vi "Func-엑셀 데이터를 그래프로 출력.vi"() -> ()   [LabVIEW 2015] (continued)
\n740.23\n740.24\n740.26\n740.28\n740.29\n740.31\n740.33\n740.34\n740.36\n740.38\n740.4\n740.41\n740.43\n740.44\n740.46\n740.48\n740.5\n740.51\n740.53\n740.54\n740.56\n740.58\n740.59\n740.61\n740.63\n740.65\n740.66\n740.68\n740.69\n740.71\n740.73\n740.74\n740.76\n740.78\n740.79\n740.81\n740.83\n740.84\n740.86\n740.88\n740.89\n740.91\n740.93\n740.94\n740.96\n740.98\n740.99\n741.01\n741.03\n741.04\n741.06\n741.08\n741.09\n741.11\n741.13\n741.14\n741.16\n741.18\n741.2\n741.21\n741.23\n741.24\n741.26\n741.28\n741.29\n741.31\n741.33\n741.34\n741.36\n741.38\n741.39\n741.41\n741.43\n741.44\n741.46\n741.48\n741.49\n741.51\n741.53\n741.54\n741.56\n741.58\n741.59\n741.61\n741.63\n741.64\n741.66\n741.68\n741.7\n741.71\n741.73\n741.74\n741.76\n741.78\n741.79\n741.81\n741.83\n741.84\n741.86\n741.88\n741.89\n741.91\n741.93\n741.94\n741.96\n741.98\n741.99\n742.01\n742.03\n742.04\n742.06\n742.08\n742.09\n742.11\n742.13\n742.14\n742.16\n742.18\n742.19\n742.21\n742.23\n742.24\n742.26\n742.28\n742.29\n742.31\n742.33\n742.34\n742.36\n742.38\n742.39\n742.41\n742.43\n742.44\n742.46\n742.48\n742.49\n742.51\n742.53\n742.54\n742.56\n742.58\n742.59\n742.61\n742.63\n742.64\n742.66\n742.68\n742.69\n742.71\n742.73\n742.74\n742.76\n742.78\n742.8\n742.81\n742.83\n742.84\n742.86\n742.88\n742.89\n742.91\n742.93\n742.94\n742.96\n742.98\n742.99\n743.01\n743.03\n743.04\n743.06\n743.08\n743.09\n743.11\n743.13\n743.15\n743.16\n743.18\n743.19\n743.21\n743.23\n743.25\n743.26\n743.28\n743.29\n743.31\n743.33\n743.34\n743.36\n743.38\n743.39\n743.41\n743.43\n743.44\n743.46\n743.48\n743.5\n743.51\n743.53\n743.54\n743.56\n743.58\n743.6\n743.61\n743.63\n743.64\n743.66\n743.68\n743.69\n743.71\n743.73\n743.74\n743.76\n743.78\n743.79\n743.81\n743.83\n743.84\n743.86\n743.88\n743.89\n743.91\n743.93\n743.95\n743.96\n743.98\n743.99\n744.01\n744.03\n744.04\n744.06\n744.08\n744.09\n744.11\n744.13\n744.14\n744.16\n744.18\n744.19\n744.21\n744.23\n744.24\n744.26\n744.28\n744.3\n744.31\n744.33\n744.34\n744.36\n744.38\n744.39\n744.41\n744.43\n744.44\n744.46\n744.48\n744.49\n744.51\n744.53\n744.54\n744.56\n744.58\n744.59\n744.61\n744.63\n744.64\n744.66\n744.68\n744.69\n744.71\n744.73\n744.74\n744.76\n744.78\n744.79\n744.81\n744.83\n744.84\n744.86\n744.88\n744.89\n744.91\n744.93\n744.94\n744.96\n744.98\n744.99\n745.01\n745.03\n745.04\n745.06\n745.08\n745.09\n745.11\n745.13\n745.14\n745.16\n745.18\n745.19\n745.21\n745.23\n745.24\n745.26\n745.28\n745.29\n745.31\n745.33\n745.34\n745.36\n745.38\n745.39\n745.41\n745.43\n745.44\n745.46\n745.48\n745.49\n745.51\n745.53\n745.54\n745.56\n745.58\n745.59\n745.61\n745.63\n745.64\n745.66\n745.68\n745.69\n745.71\n745.73\n745.74\n745.76\n745.78\n745.79\n745.81\n745.83\n745.84\n745.86\n745.88\n745.89\n745.91\n745.93\n745.94\n745.96\n745.98\n745.99\n746.01\n746.03\n746.04\n746.06\n746.08\n746.09\n746.11\n746.13\n746.14\n746.16\n746.18\n746.19\n746.21\n746.23\n746.25\n746.26\n746.28\n746.29\n746.31\n746.33\n746.34\n746.36\n746.38\n746.39\n746.41\n746.43\n746.44\n746.46\n746.48\n746.5\n746.51\n746.53\n746.54\n746.56\n746.58\n746.6\n746.61\n746.63\n746.64\n746.66\n746.68\n746.69\n746.71\n746.73\n746.74\n746.76\n746.78\n746.79\n746.81\n746.83\n746.84\n746.86\n746.88\n746.89\n746.91\n746.93\n746.94\n746.96\n746.98\n746.99\n747.01\n747.03\n747.05\n747.06\n747.08\n747.09\n747.11\n747.13\n747.14\n747.16\n747.18\n747.19\n747.21\n747.23\n747.24\n747.26\n747.28\n747.29\n747.31\n747.33\n747.34\n747.36\n747.38\n747.39\n747.41\n747.43\n747.44\n747.46\n747.48\n747.49\n747.51\n747.53\n747.54\n747.56\n747.58\n747.59\n747.61\n747.63\n747.64\n747.66\n747.68\n747.69\n747.71\n747.73\n747.74\n747.76\n747.78\n747.79\n747.81\n747.83\n747.84\n747.86\n747.88\n747.9\n747.91\n747.93\n747.94\n747.96\n747.98\n747.99\n748.01\n748.03\n748.04\n748.06\n748.08\n748.09\n748.11\n748.13\n748.14\n748.16\n748.18\n748.19\n748.21\n748.23\n748.24\n748.26\n748.28\n748.29\n748.31\n748.33\n748.34\n748.36\n748.38\n748.39\n748.41\n748.43\n748.44\n748.46\n748.48\n748.49\n748.51\n748.53\n748.54\n748.56\n748.58\n748.59\n748.61\n748.63\n748.64\n748.66\n748.68\n748.69\n748.71\n748.73\n748.74\n748.76\n748.78\n748.79\n748.81\n748.83\n748.84\n748.86\n748.88\n748.89\n748.91\n748.93\n748.94\n748.96\n748.98\n749\n749.01\n749.03\n749.04\n749.06\n749.08\n749.09\n749.11\n749.13\n749.14\n749.16\n749.18\n749.19\n749.21\n749.23\n749.24\n749.26\n749.28\n749.29\n749.31\n749.33\n749.35\n749.36\n749.38\n749.39\n749.41\n749.43\n749.44\n749.46\n749.48\n749.49\n749.51\n749.53\n749.54\n749.56\n749.58\n749.6\n749.61\n749.63\n749.64\n749.66\n749.68\n749.7\n749.71\n749.73\n749.74\n749.76\n749.78\n749.79\n749.81\n749.83\n749.85\n749.86\n749.88\n749.89\n749.91\n749.93\n749.95\n749.96\n749.98\n749.99\n750.01\n750.03\n750.05\n750.06\n750.08\n750.09\n750.11\n750.13\n750.14\n750.16\n750.18\n750.19\n750.21\n750.23\n750.24\n750.26\n750.28\n750.3\n750.31\n750.33\n750.34\n750.36\n750.38\n750.39\n750.41\n750.43\n750.44\n750.46\n750.48\n750.49\n750.51\n750.53\n750.54\n750.56\n750.58\n750.59\n750.61\n750.63\n750.64\n750.66\n750.68\n750.69\n750.71\n750.73\n750.74\n750.76\n750.78\n750.79\n750.81\n750.83\n750.84\n750.86\n750.88\n750.89\n750.91\n750.93\n750.94\n750.96\n750.98\n750.99\n751.01\n751.03\n751.04\n751.06\n751.08\n751.09\n751.11\n751.13\n751.14\n751.16\n751.18\n751.19\n751.21\n751.23\n751.24\n751.26\n751.28\n751.29\n751.31\n751.33\n751.34\n751.36\n751.38\n751.39\n751.41\n751.43\n751.44\n751.46\n751.48\n751.49\n751.51\n751.53\n751.54\n751.56\n751.58\n751.59\n751.61\n751.63\n751.64\n751.66\n751.68\n751.69\n751.71\n751.73\n751.74\n751.76\n751.78\n751.79\n751.81\n751.83\n751.84\n751.86\n751.88\n751.89\n751.91\n751.93\n751.94\n751.96\n751.98\n751.99\n752.01\n752.03\n752.04\n752.06\n752.08\n752.1\n752.11\n752.13\n752.14\n752.16\n752.18\n752.19\n752.21\n752.23\n752.24\n752.26\n752.28\n752.29\n752.31\n752.33\n752.35\n752.36\n752.38\n752.39\n752.41\n752.43\n752.45\n752.46\n752.48\n752.49\n752.51\n752.53\n752.54\n752.56\n752.58\n752.59\n752.61\n752.63\n752.64\n752.66\n752.68\n752.7\n752.71\n752.73\n752.74\n752.76\n752.78\n752.8\n752.81\n752.83\n752.84\n752.86\n752.88\n752.89\n752.91\n752.93\n752.94\n752.96\n752.98\n752.99\n753.01\n753.03\n753.05\n753.06\n753.08\n753.09\n753.11\n753.13\n753.14\n753.16\n753.18\n753.19\n753.21\n753.23\n753.24\n753.26\n753.28\n753.29\n753.31\n753.33\n753.34\n753.36\n753.38\n753.4\n753.41\n753.43\n753.44\n753.46\n753.48\n753.49\n753.51\n753.53\n753.54\n753.56\n753.58\n753.59\n753.61\n753.63\n753.65\n753.66\n753.68\n753.69\n753.71\n753.73\n753.75\n753.76\n753.78\n753.79\n753.81\n753.83\n753.84\n753.86\n753.88\n753.89\n753.91\n753.93\n753.95\n753.96\n753.98\n753.99\n754.01\n754.03\n754.04\n754.06\n754.08\n754.09\n754.11\n754.13\n754.14\n754.16\n754.18\n754.19\n754.21\n754.23\n754.24\n754.26\n754.28\n754.29\n754.31\n754.33\n754.34\n754.36\n754.38\n754.39\n754.41\n754.43\n754.44\n754.46\n754.48\n754.49\n754.51\n754.53\n754.54\n754.56\n754.58\n754.59\n754.61\n754.63\n754.64\n754.66\n754.68\n754.69\n754.71\n754.73\n754.74\n754.76\n754.78\n754.79\n754.81\n754.83\n754.84\n754.86\n754.88\n754.89\n754.91\n754.93\n754.94\n754.96\n754.98\n754.99\n755.01\n755.03\n755.04\n755.06\n755.08\n755.1\n755.11\n755.13\n755.14\n755.16\n755.18\n755.19\n755.21\n755.23\n755.24\n755.26\n755.28\n755.29\n755.31\n755.33\n755.34\n755.36\n755.38\n755.39\n755.41\n755.43\n755.45\n755.46\n755.48\n755.49\n755.51\n755.53\n755.54\n755.56\n755.58\n755.59\n755.61\n755.63\n755.64\n755.66\n755.68\n755.69\n755.71\n755.73\n755.74\n755.76\n755.78\n755.8\n755.81\n755.83\n755.84\n755.86\n755.88\n755.9\n755.91\n755.93\n755.94\n755.96\n755.98\n755.99\n756.01\n756.03\n756.05\n756.06\n756.08\n756.09\n756.11\n756.13\n756.14\n756.16\n756.18\n756.19\n756.21\n756.23\n756.24\n756.26\n756.28\n756.29\n756.31\n756.33\n756.34\n756.36\n756.38\n756.4\n756.41\n756.43\n756.44\n756.46\n756.48\n756.49\n756.51\n756.53\n756.54\n756.56\n756.58\n756.59\n756.61\n756.63\n756.65\n756.66\n756.68\n756.69\n756.71\n756.73\n756.74\n756.76\n756.78\n756.79\n756.81\n756.83\n756.84\n756.86\n756.88\n756.89\n756.91\n756.93\n756.94\n756.96\n756.98\n756.99\n757.01\n757.03\n757.04\n757.06\n757.08\n757.09\n757.11\n757.13\n757.14\n757.16\n757.18\n757.19\n757.21\n757.23\n757.24\n757.26\n757.28\n757.29\n757.31\n757.33\n757.34\n757.36\n757.38\n757.39\n757.41\n757.43\n757.44\n757.46\n757.48\n757.49\n757.51\n757.53\n757.54\n757.56\n757.58\n757.59\n757.61\n757.63\n757.64\n757.66\n757.68\n757.69\n757.71\n757.73\n757.74\n757.76\n757.78\n757.79\n757.81\n757.83\n757.84\n757.86\n757.88\n757.89\n757.91\n757.93\n757.94\n757.96\n757.98\n757.99\n758.01\n758.03\n758.04\n758.06\n758.08\n758.09\n758.11\n758.13\n758.14\n758.16\n758.18\n758.2\n758.21\n758.23\n758.24\n758.26\n758.28\n758.29\n758.31\n758.33\n758.34\n758.36\n758.38\n758.39\n758.41\n758.43\n758.44\n758.46\n758.48\n758.49\n758.51\n758.53\n758.55\n758.56\n758.58\n758.59\n758.61\n758.63\n758.64\n758.66\n758.68\n758.69\n758.71\n758.73\n758.74\n758.76\n758.78\n758.8\n758.81\n758.83\n758.84\n758.86\n758.88\n758.9\n758.91\n758.93\n758.94\n758.96\n758.98\n758.99\n759.01\n759.03\n759.04\n759.06\n759.08\n759.09\n759.11\n759.13\n759.15\n759.16\n759.18\n759.19\n759.21\n759.23\n759.25\n759.26\n759.28\n759.29\n759.31\n759.33\n759.34\n759.36\n759.38\n759.39\n759.41\n759.43\n759.44\n759.46\n759.48\n759.5\n759.51\n759.53\n759.54\n759.56\n759.58\n759.59\n759.61\n759.63\n759.64\n759.66\n759.68\n759.7\n759.71\n759.73\n759.74\n759.76\n759.78\n759.79\n759.81\n759.83\n759.84\n759.86\n759.88\n759.89\n759.91\n759.93\n759.94\n759.96\n759.98\n759.99\n760.01\n760.03\n760.04\n760.06\n760.08\n760.09\n760.11\n760.13\n760.14\n760.16\n760.18\n760.19\n760.21\n760.23\n760.24\n760.26\n760.28\n760.29\n760.31\n760.33\n760.34\n760.36\n760.38\n760.39\n760.41\n760.43\n760.44\n760.46\n760.48\n760.49\n760.51\n760.53\n760.54\n760.56\n760.58\n760.59\n760.61\n760.63\n760.64\n760.66\n760.68\n760.69\n760.71\n760.73\n760.74\n760.76\n760.78\n760.79\n760.81\n760.83\n760.84\n760.86\n760.88\n760.89\n760.91\n760.93\n760.94\n760.96\n760.98\n760.99\n761.01\n761.03\n761.04\n761.06\n761.08\n761.09\n761.11\n761.13\n761.14\n761.16\n761.18\n761.19\n761.21\n761.23\n761.24\n761.26\n761.28\n761.29\n761.31\n761.33\n761.34\n761.36\n761.38\n761.39\n761.41\n761.43\n761.44\n761.46\n761.48\n761.49\n761.51\n761.53\n761.54\n761.56\n761.58\n761.59\n761.61\n761.63\n761.65\n761.66\n761.68\n761.69\n761.71\n761.73\n761.74\n761.76\n761.78\n761.79\n761.81\n761.83\n761.84\n761.86\n761.88\n761.9\n761.91\n761.93\n761.94\n761.96\n761.98\n762\n762.01\n762.03\n762.04\n762.06\n762.08\n762.09\n762.11\n762.13\n762.14\n762.16\n762.18\n762.19\n762.21\n762.23\n762.25\n762.26\n762.28\n762.29\n762.31\n762.33\n762.34\n762.36\n762.38\n762.39\n762.41\n762.43\n762.45\n762.46\n762.48\n762.49\n762.51\n762.53\n762.54\n762.56\n762.58\n762.59\n762.61\n762.63\n762.64\n762.66\n762.68\n762.69\n762.71\n762.73\n762.74\n762.76\n762.78\n762.79\n762.81\n762.83\n762.84\n762.86\n762.88\n762.89\n762.91\n762.93\n762.95\n762.96\n762.98\n762.99\n763.01\n763.03\n763.04\n763.06\n763.08\n763.09\n763.11\n763.13\n763.14\n763.16\n763.18\n763.19\n763.21\n763.23\n763.24\n763.26\n763.28\n763.29\n763.31\n763.33\n763.34\n763.36\n763.38\n763.39\n763.41\n763.43\n763.44\n763.46\n763.48\n763.49\n763.51\n763.53\n763.54\n763.56\n763.58\n763.59\n763.61\n763.63\n763.64\n763.66\n763.68\n763.69\n763.71\n763.73\n763.74\n763.76\n763.78\n763.79\n763.81\n763.83\n763.84\n763.86\n763.88\n763.89\n763.91\n763.93\n763.94\n763.96\n763.98\n763.99\n764.01\n764.03\n764.04\n764.06\n764.08\n764.09\n764.11\n764.13\n764.14\n764.16\n764.18\n764.19\n764.21\n764.23\n764.24\n764.26\n764.28\n764.29\n764.31\n764.33\n764.34\n764.36\n764.38\n764.39\n764.41\n764.43\n764.44\n764.46\n764.48\n764.49\n764.51\n764.53\n764.54\n764.56\n764.58\n764.59\n764.61\n764.63\n764.65\n764.66\n764.68\n764.69\n764.71\n764.73\n764.75\n764.76\n764.78\n764.79\n764.81\n764.83\n764.84\n764.86\n764.88\n764.89\n764.91\n764.93\n764.94\n764.96\n764.98\n765\n765.01\n765.03\n765.04\n765.06\n765.08\n765.1\n765.11\n765.13\n765.14\n765.16\n765.18\n765.19\n765.21\n765.23\n765.25\n765.26\n765.28\n765.29\n765.31\n765.33\n765.35\n765.36\n765.38\n765.39\n765.41\n765.43\n765.45\n765.46\n765.48\n765.49\n765.51\n765.53\n765.54\n765.56\n765.58\n765.59\n765.61\n765.63\n765.64\n765.66\n765.68\n765.69\n765.71\n765.73\n765.74\n765.76\n765.78\n765.79\n765.81\n765.83\n765.84\n765.86\n765.88\n765.89\n765.91\n765.93\n765.95\n765.96\n765.98\n765.99\n766.01\n766.03\n766.04\n766.06\n766.08\n766.09\n766.11\n766.13\n766.14\n766.16\n766.18\n766.19\n766.21\n766.23\n766.24\n766.26\n766.28\n766.3\n766.31\n766.33\n766.34\n766.36\n766.38\n766.39\n766.41\n766.43\n766.44\n766.46\n766.48\n766.49\n766.51\n766.53\n766.54\n766.56\n766.58\n766.59\n766.61\n766.63\n766.64\n766.66\n766.68\n766.69\n766.71\n766.73\n766.74\n766.76\n766.78\n766.79\n766.81\n766.83\n766.84\n766.86\n766.88\n766.89\n766.91\n766.93\n766.94\n766.96\n766.98\n766.99\n767.01\n767.03\n767.04\n767.06\n767.08\n767.09\n767.11\n767.13\n767.14\n767.16\n767.18\n767.19\n767.21\n767.23\n767.24\n767.26\n767.28\n767.29\n767.31\n767.33\n767.34\n767.36\n767.38\n767.39\n767.41\n767.43\n767.44\n767.46\n767.48\n767.49\n767.51\n767.53\n767.54\n767.56\n767.58\n767.59\n767.61\n767.63\n767.64\n767.66\n767.68\n767.69\n767.71\n767.73\n767.75\n767.76\n767.78\n767.79\n767.81\n767.83\n767.84\n767.86\n767.88\n767.89\n767.91\n767.93\n767.94\n767.96\n767.98\n767.99\n768.01\n768.03\n768.04\n768.06\n768.08\n768.1\n768.11\n768.13\n768.14\n768.16\n768.18\n768.19\n768.21\n768.23\n768.24\n768.26\n768.28\n768.29\n768.31\n768.33\n768.35\n768.36\n768.38\n768.39\n768.41\n768.43\n768.45\n768.46\n768.48\n768.49\n768.51\n768.53\n768.54\n768.56\n768.58\n768.59\n768.61\n768.63\n768.64\n768.66\n768.68\n768.69\n768.71\n768.73\n768.74\n768.76\n768.78\n768.79\n768.81\n768.83\n768.84\n768.86\n768.88\n768.89\n768.91\n768.93\n768.94\n768.96\n768.98\n768.99\n769.01\n769.03\n769.04\n769.06\n769.08\n769.09\n769.11\n769.13\n769.14\n769.16\n769.18\n769.19\n769.21\n769.23\n769.24\n769.26\n769.28\n769.29\n769.31\n769.33\n769.34\n769.36\n769.38\n769.39\n769.41\n769.43\n769.44\n769.46\n769.48\n769.49\n769.51\n769.53\n769.54\n769.56\n769.58\n769.6\n769.61\n769.63\n769.64\n769.66\n769.68\n769.69\n769.71\n769.73\n769.74\n769.76\n769.78\n769.79\n769.81\n769.83\n769.84\n769.86\n769.88\n769.89\n769.91\n769.93\n769.94\n769.96\n769.98\n769.99\n770.01\n770.03\n770.04\n770.06\n770.08\n770.09\n770.11\n770.13\n770.14\n770.16\n770.18\n770.19\n770.21\n770.23\n770.24\n770.26\n770.28\n770.29\n770.31\n770.33\n770.34\n770.36\n770.38\n770.39\n770.41\n770.43\n770.44\n770.46\n770.48\n770.49\n770.51\n770.53\n770.54\n770.56\n770.58\n770.59\n770.61\n770.63\n770.64\n770.66\n770.68\n770.69\n770.71\n770.73\n770.74\n770.76\n770.78\n770.79\n770.81\n770.83\n770.85\n770.86\n770.88\n770.89\n770.91\n770.93\n770.94\n770.96\n770.98\n770.99\n771.01\n771.03\n771.04\n771.06\n771.08\n771.09\n771.11\n771.13\n771.14\n771.16\n771.18\n771.2\n771.21\n771.23\n771.24\n771.26\n771.28\n771.29\n771.31\n771.33\n771.34\n771.36\n771.38\n771.39\n771.41\n771.43\n771.45\n771.46\n771.48\n771.49\n771.51\n771.53\n771.55\n771.56\n771.58\n771.59\n771.61\n771.63\n771.64\n771.66\n771.68\n771.7\n771.71\n771.73\n771.74\n771.76\n771.78\n771.79\n771.81\n771.83\n771.84\n771.86\n771.88\n771.9\n771.91\n771.93\n771.94\n771.96\n771.98\n771.99\n772.01\n772.03\n772.04\n772.06\n772.08\n772.09\n772.11\n772.13\n772.14\n772.16\n772.18\n772.19\n772.21\n772.23\n772.24\n772.26\n772.28\n772.29\n772.31\n772.33\n772.34\n772.36\n772.38\n772.39\n772.41\n772.43\n772.44\n772.46\n772.48\n772.49\n772.51\n772.53\n772.54\n772.56\n772.58\n772.6\n772.61\n772.63\n772.64\n772.66\n772.68\n772.69\n772.71\n772.73\n772.74\n772.76\n772.78\n772.79\n772.81\n772.83\n772.84\n772.86\n772.88\n772.89\n772.91\n772.93\n772.94\n772.96\n772.98\n772.99\n773.01\n773.03\n773.04\n773.06\n773.08\n773.09\n773.11\n773.13\n773.14\n773.16\n773.18\n773.19\n773.21\n773.23\n773.24\n773.26\n773.28\n773.29\n773.31\n773.33\n773.34\n773.36\n773.38\n773.39\n773.41\n773.43\n773.44\n773.46\n773.48\n773.49\n773.51\n773.53\n773.54\n773.56\n773.58\n773.6\n773.61\n773.63\n773.64\n773.66\n773.68\n773.69\n773.71\n773.73\n773.74\n773.76\n773.78\n773.79\n773.81\n773.83\n773.84\n773.86\n773.88\n773.89\n773.91\n773.93\n773.95\n773.96\n773.98\n773.99\n774.01\n774.03\n774.04\n774.06\n774.08\n774.09\n774.11\n774.13\n774.14\n774.16\n774.18\n774.2\n774.21\n774.23\n774.24\n774.26\n774.28\n774.3\n774.31\n774.33\n774.34\n774.36\n774.38\n774.39\n774.41\n774.43\n774.44\n774.46\n774.48\n774.49\n774.51\n774.53\n774.55\n774.56\n774.58\n774.59\n774.61\n774.63\n774.65\n774.66\n774.68\n791.65\n791.81\n791.98\n792.15\n792.31\n792.48\n792.65\n792.81\n792.98\n793.15\n793.31\n793.48\n793.65\n793.81\n793.98\n794.15\n794.31\n794.48\n794.65\n794.81\n794.98\n795.15\n795.31\n795.48\n795.65\n795.81\n795.98\n796.15\n796.32\n796.48\n796.65\n796.81\n796.98\n797.15\n797.31\n797.48\n797.65\n797.81\n797.98\n798.15\n798.31\n798.48\n798.65\n798.81\n798.98\n799.15\n799.31\n799.48\n799.65\n799.81\n799.98\n800.15\n800.31\n800.48\n800.65\n800.81\n800.98\n801.15\n801.32\n801.48\n801.65\n801.81\n801.98\n802.15\n802.31\n802.48\n802.65\n802.81\n802.98\n803.15\n803.31\n803.48\n803.65\n803.81\n803.98\n804.15\n804.32\n804.48\n804.65\n804.81\n804.98\n805.15\n805.31\n805.48\n805.65\n805.81\n805.98\n806.15\n806.31\n806.48\n806.65\n806.81\n806.98\n807.15\n807.32\n807.48\n807.65\n807.81\n807.98\n808.15\n808.31\n808.48\n808.65\n808.81\n808.98\n809.15\n809.31\n809.48\n809.65\n809.82\n809.98\n810.15\n810.31\n810.48\n810.65\n810.81\n810.98\n811.15\n811.31\n811.48\n811.65\n811.81\n811.98\n812.15\n812.31\n812.48\n812.65\n812.81\n812.98\n813.15\n813.31\n813.48\n813.65\n813.81\n813.98\n814.15\n814.31\n814.48\n814.65\n814.82\n814.98\n815.15\n815.31\n815.48\n815.65\n815.81\n815.98\n816.15\n816.31\n816.48\n816.65\n816.81\n816.98\n817.15\n817.31\n817.48\n817.65\n817.81\n817.98\n818.15\n818.31\n818.48\n818.65\n818.81\n818.98\n819.15\n819.31\n819.48\n819.65\n819.81\n819.98\n820.15\n820.32\n820.48\n820.65\n820.81\n820.98\n821.15\n821.31\n821.51\n821.65\n821.82\n821.98\n822.15\n822.31\n822.48\n822.65\n822.82\n822.98\n823.15\n823.31\n823.48\n823.65\n823.81\n823.98\n824.15\n824.31\n824.48\n824.65\n824.81\n824.98\n825.15\n825.31\n825.48\n825.65\n825.82\n825.98\n826.15\n826.31\n826.48\n826.66\n826.82\n826.99\n827.16\n827.32\n827.49\n827.66\n827.82\n827.99\n828.16\n828.32\n828.49\n828.66\n828.82\n828.99\n829.16\n829.32\n829.49\n829.66\n829.82\n829.99\n830.16\n830.32\n830.49\n830.66\n830.83\n831\n831.16\n831.33\n831.5\n831.65\n831.66\n831.68\n831.69\n831.71\n831.73\n831.75\n831.76\n831.78\n831.79\n831.81\n831.83\n831.84\n831.86\n831.88\n831.9\n831.91\n831.93\n831.94\n831.96\n831.98\n831.99\n832.01\n832.03\n832.04\n832.06\n832.08\n832.09\n832.11\n832.13\n832.14\n832.16\n832.18\n832.19\n832.21\n832.23\n832.24\n832.26\n832.28\n832.29\n832.31\n832.33\n832.34\n832.36\n832.38\n832.39\n832.41\n832.43\n832.44\n832.46\n832.48\n832.49\n832.51\n832.53\n832.54\n832.56\n832.58\n832.59\n832.61\n832.63\n832.64\n832.66\n832.68\n832.69\n832.71\n832.73\n832.74\n832.76\n832.78\n832.79\n832.81\n832.83\n832.84\n832.86\n832.88\n832.89\n832.91\n832.93\n832.94\n832.96\n832.98\n832.99\n833.01\n833.03\n833.04\n833.06\n833.08\n833.09\n833.11\n833.13\n833.14\n833.16\n833.18\n833.19\n833.21\n833.23\n833.24\n833.26\n833.28\n833.29\n833.31\n833.33\n833.34\n833.36\n833.38\n833.39\n833.41\n833.43\n833.44\n833.46\n833.48\n833.49\n833.51\n833.53\n833.54\n833.56\n833.58\n833.59\n833.61\n833.63\n833.64\n833.66\n833.68\n833.69\n833.71\n833.73\n833.74\n833.76\n833.78\n833.79\n833.81\n833.83\n833.84\n833.86\n833.88\n833.89\n833.91\n833.93\n833.94\n833.96\n833.98\n833.99\n834.01\n834.03\n834.05\n834.06\n834.08\n834.09\n834.11\n834.13\n834.14\n834.16\n834.18\n834.19\n834.21\n834.23\n834.24\n834.26\n834.28\n834.29\n834.31\n834.33\n834.34\n834.36\n834.38\n834.4\n834.41\n834.43\n834.44\n834.46\n834.48\n834.49\n834.51\n834.53\n834.54\n834.56\n834.58\n834.59\n834.61\n834.63\n834.64\n834.66\n834.68\n834.69\n834.71\n834.73\n834.75\n834.76\n834.78\n834.79\n834.81\n834.83\n834.85\n834.86\n834.88\n834.89\n834.91\n834.93\n834.94\n
